vi "Bit Shift Out.vi"(7 "output enable":bool, 9 "reset":bool, 10 "shift bits":bool, 11 "sample":u32) -> (3 "bit out":bool)   [LabVIEW 2013, in "I2S-TDM.lvlib"]
uses:
  I2S-TDM.lvlib
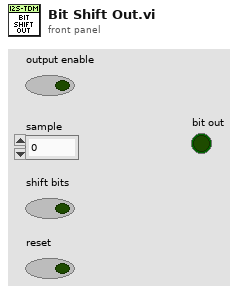
[diagram p1: front panel]
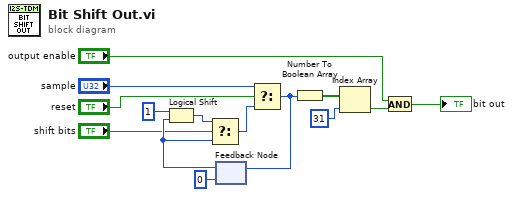
[diagram p0: block diagram]
diagram:
  n1 = feedback #1(u32 0) -> (w4:u32)
  n2 = Logical Shift(y=i16 1, x=w4) -> (x << y=w11:u32)
  n3 = Select(t=w11, s="shift bits", f=w4) -> (s? t:f=w3:u32)
  n4 = Select(t="sample", s="reset", f=w3) -> (s? t:f=w1:u32)
  n5 = feedback-in #1(w1) -> ()
  n6 = Number To Boolean Array(number=w1) -> (Boolean array=w7:bool[])
  n7 = Index Array(array=w7, index=31) -> (element=w5:bool)
  n8 = And(x="output enable", y=w5) -> (x .and. y?=→"bit out":bool)
